vi "Write iCalendar File.vi"(7 "Recipient's Email Address":T1, 8 "error in":errorcluster, 10 "iCalendar File Configuration":T2={"File Name"="", "Orginizer Name"="", "Organizer email"="", "Subject"="", "Location"="yerevan", "Start Date and Time "=timestamp(3579138000 s since 1904-01-01), "End Date and Time"=timestamp(3579148800 s since 1904-01-01)}, 11 "Path to Save":path) -> (0 "error out":errorcluster, 3 "Path Out":path)   [LabVIEW 2016]
doc: "Write iCalendar File VI creates an iCalendar file based on the inputs."
uses:
  controls/ics File Configuration.ctl
  controls/Receipants Email Address.ctl
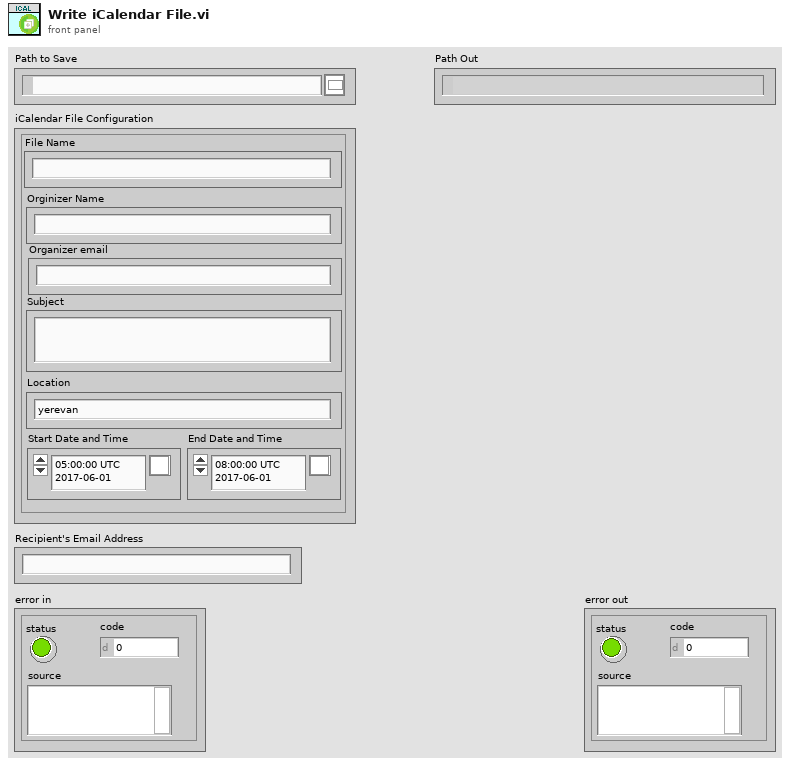
[diagram p1: front panel]
types:
  T1 = typedef "Receipants Email Address.ctl" = string
  T2 = typedef "ics File Configuration.ctl" = cluster{"File Name":string, "Orginizer Name":string, "Organizer email":string, "Subject":string, "Location":string, "Start Date and Time ":timestamp, "End Date and Time":timestamp}
  T3 = enum16{"open", "replace", "create", "open or create", "replace or create", "replace or create with confirmation"}
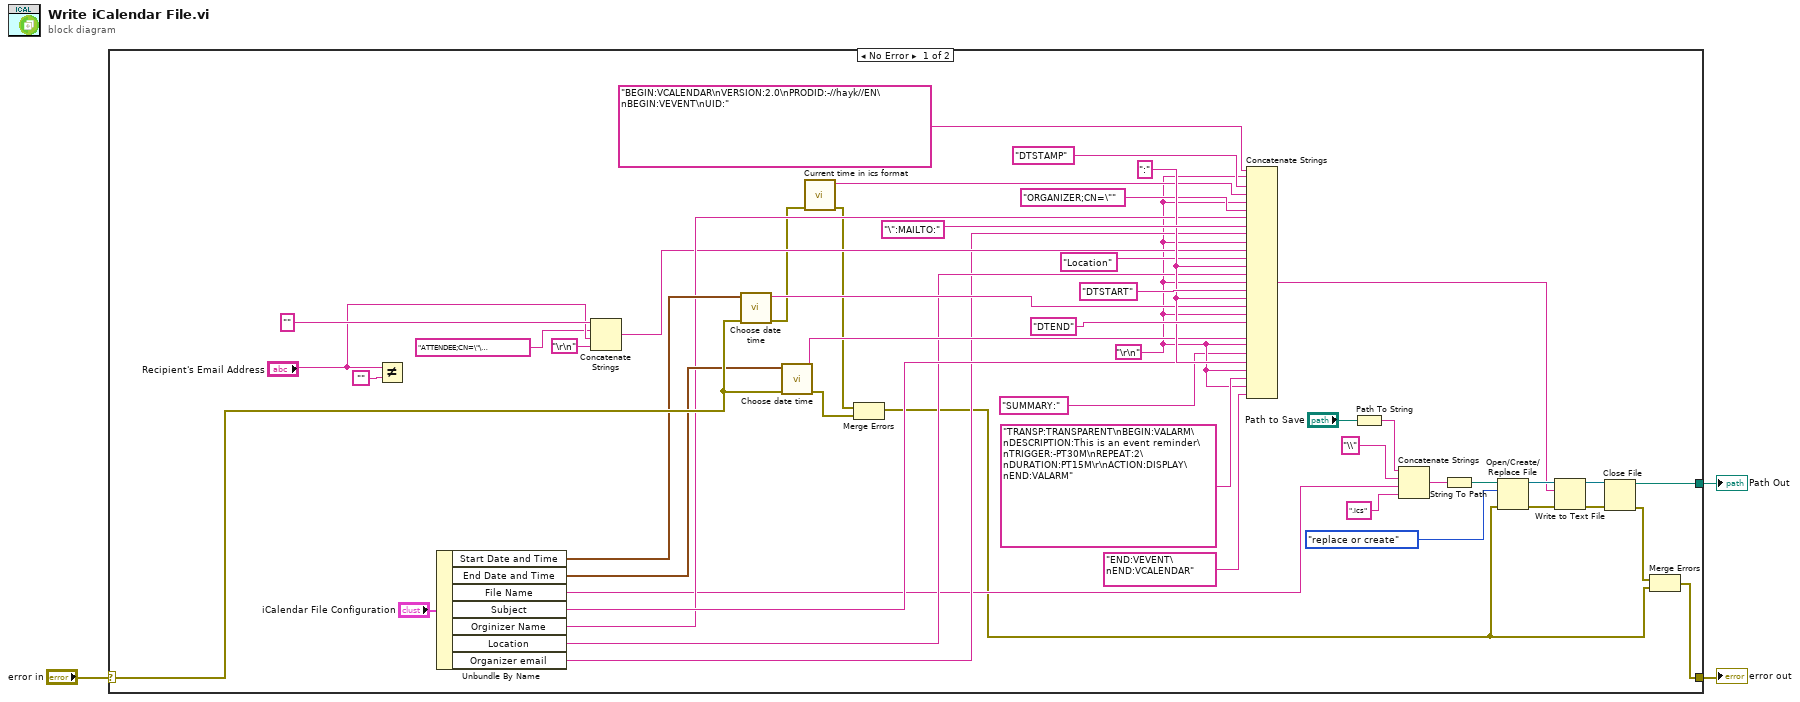
[diagram p0: block diagram]
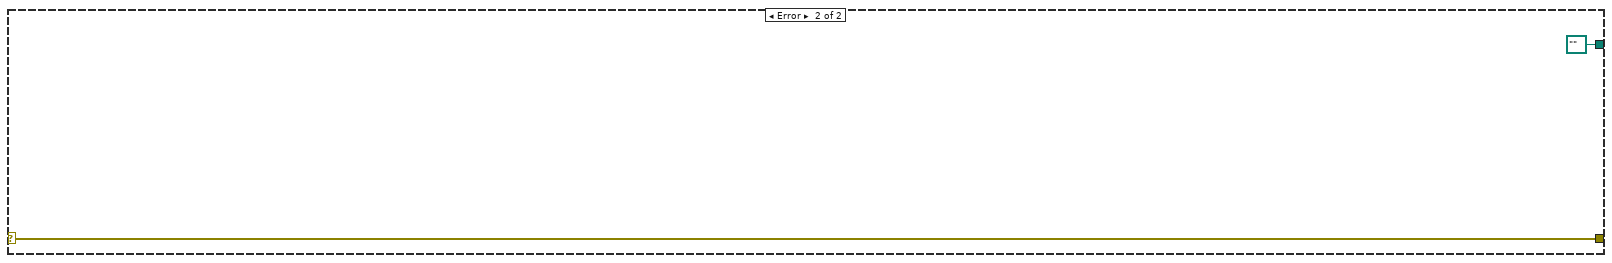
[diagram p2: hidden frame]
diagram:
  n1 = case shown="No Error" "error in" {
    selector: "error in" -> [w41 w54]
    tunnel: [w8 w54] -> w3
    tunnel: [w7 path "" ("path")] -> w1
    frame No Error {
      w45 = ":" ("string")
      w27 = "\r\n"
      n2 = Not Equal?(x="Recipient's Email Address", y="") -> ()  [unwired: 1 out]
      n3 = Unbundle By Name("iCalendar File Configuration") -> ("Start Date and Time"=w39:timestamp, "End Date and Time"=w38:timestamp, "File Name"=w6:string, "Subject"=w37:string, "Orginizer Name"=w36:string, "Location"=w35:string, "Organizer email"=w28:string)
      n4 = Concatenate Strings("", "ATTENDEE;CN=\"\";RSVP=TRUE:" ("string"), "Recipient's Email Address", "\r\n") -> (w31:string)
      n5 = call "Choose date time.vi"("Error In"=w41, "Time"=w39) -> ("Error Out"=w25:errorcluster, "ics format Date/Time"=w43:string)  [unwired: 8 in]
      n6 = call "Choose date time.vi"("Error In"=w41, "Time"=w38) -> ("Error Out"=w34:errorcluster, "ics format Date/Time"=w44:string)  [unwired: 8 in]
      n7 = call "Current time in ics format.vi"("Error In"=w25) -> ("Error Out"=w24:errorcluster, "current time"=w42:string)  [unwired: 9 in]
      n8 = Merge Errors(w24, w34) -> (w5:errorcluster)
      n9 = Concatenate Strings("BEGIN:VCALENDAR\nVERSION:2.0\nPRODID:-//hayk//EN\nBEGIN:VEVENT\nUID:", w27, "DTSTAMP", w42, w27, "ORGANIZER;CN=\"" ("string"), w36, "\":MAILTO:" ("string"), w28, w27, w31, "Location" ("string"), w45, w35, w27, "DTSTART" ("string"), w45, w43, w27, "DTEND" ("string"), w45, w44, w27, "SUMMARY:" ("string"), w37, w27, "TRANSP:TRANSPARENT\nBEGIN:VALARM\nDESCRIPTION:This is an event reminder\nTRIGGER:-PT30M\nREPEAT:2\nDURATION:PT15M\r\nACTION:DISPLAY\nEND:VALARM" ("string"), w27, "END:VEVENT\nEND:VCALENDAR" ("string")) -> (w12:string)
      n10 = Path To String(path="Path to Save") -> (string=w18:string)
      n11 = Concatenate Strings(w18, "\\" ("string"), w6, ".ics" ("string")) -> (w19:string)
      n12 = String To Path(string=w19) -> (path=w20:path)
      n13 = Open/Create/Replace File(file path (use dialog)=w20, error in=w5, operation (0:open)=T3."replace or create") -> (refnum out=w16:refnum<file>, error out=w17:errorcluster)  [unwired: 3 in, 1 out]
      n14 = Write to Text File(file (use dialog)=w16, text=w12, error in=w17) -> (refnum out=w11:refnum<file>, error out=w10:errorcluster)  [unwired: 1 in, 1 out]
      n15 = Close File(refnum=w11, error in=w10) -> (path=w7:path, error out=w9:errorcluster)
      n16 = Merge Errors(w9, w5) -> (w8:errorcluster)
    }
    frame Error {
    }
  }
  "error out" <- w3
  "Path Out" <- w1
